vi "TW Update VI name.vi"(8 "error in":errorcluster, 9 "VI Name":string="Test UI.vi", 10 "Project Name":string, 11 "Name to VI Map in":map{string, refnum<vi>}(c390)) -> (0 "error out":errorcluster, 3 "Name to VI Map out":map{string, refnum<vi>}(c390))   [LabVIEW 2021, in "Plugin Generator.lvlib"]
uses:
  Plugin Generator.lvlib
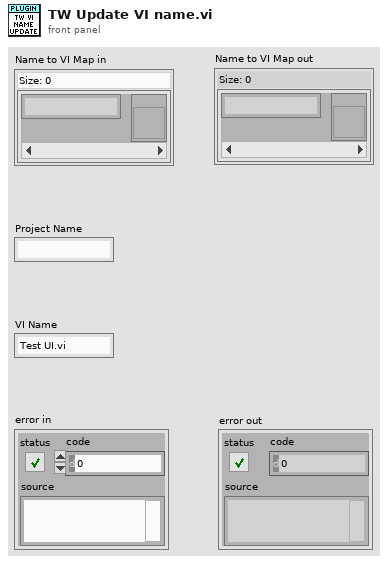
[diagram p1: front panel]
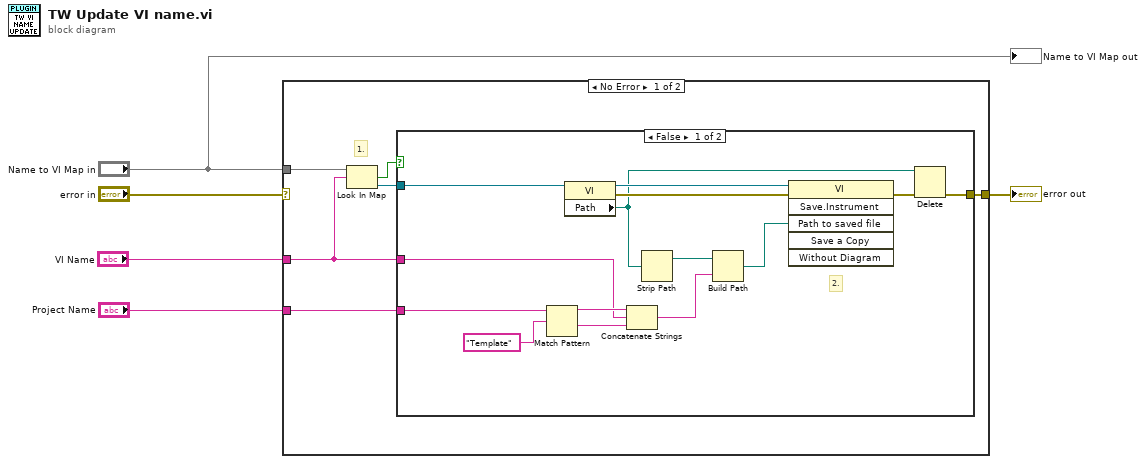
[diagram p0: block diagram]
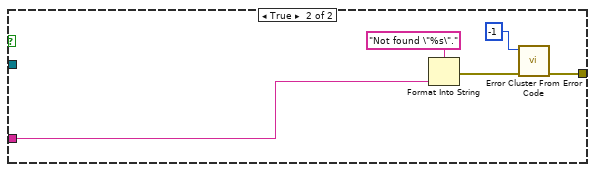
[diagram p2: hidden frame]
diagram:
  n1 = case shown="No Error" "error in" {
    selector: "error in" -> [_ w31]
    tunnel: "Project Name" -> [w11 _]
    tunnel: [w10 w31] -> w4
    tunnel: "Name to VI Map in" -> [w9 _]
    tunnel: "VI Name" -> [w6 _]
    frame No Error {
      # "1."
      n2 = Look In Map(map=w9, key=w6) -> (key not found?=w7:bool, value=w8:refnum<vi>)  [unwired: 1 in]
      n3 = case shown="False" w7 {
        tunnel: w11 -> [w17 _]
        tunnel: [w20 w29] -> w10
        tunnel: w8 -> [w18 _]
        tunnel: w6 -> [w12 w26]
        frame False {
          # "2."
          n4 = Match Pattern(string=w17, regular expression="Template") -> (before substring=w15:string, after substring=w14:string)  [unwired: 1 in, 2 out]
          n5 = property class="VI"(reference=w18) -> (reference out=w25:refnum<vi>, error out=w22:errorcluster, "Path"=w19:path)  [unwired: 1 in]
          n6 = Concatenate Strings(w15, w12, w14) -> (w13:string)
          n7 = Strip Path(path=w19) -> (stripped path=w23:path)  [unwired: 1 out]
          n8 = Build Path(base path=w23, name or relative path=w13) -> (appended path=w24:path)
          n9 = invoke class="VI" method="Save.Instrument"(reference=w25, error in=w22, "Path to saved file"=w24) -> (error out=w21:errorcluster)  [unwired: 3 in, 5 out]
          n10 = Delete(path (use dialog)=w19, error in=w21) -> (error out=w20:errorcluster)  [unwired: 3 in, 2 out]
        }
        frame True {
          n11 = Format Into String(format string="Not found \"%s\"." ("error message (\"\")"), w26) -> (error out=w27:errorcluster)  [unwired: 2 in, 1 out]
          n12 = call <vilib>:"Error Cluster From Error Code.vi"("error in (no error)"=w27, "error code (0)"=-1) -> ("error out"=w29:errorcluster)  [unwired: 7 in]
        }
      }
    }
    frame Error {
    }
  }
  "error out" <- w4
  "Name to VI Map out" <- "Name to VI Map in"
